vi "WriteBitDepth.vi"(8 "error in":errorcluster, 10 "BitDepth":u32, 11 "Image Reference In":T1) -> (0 "error out":errorcluster, 3 "Image Reference Out":T1)   [LabVIEW 2024, in "OpenLvVision_Image.lvlib" / "Management.lvlib"]
doc: "Sets number of bits per pixel, determining the range of representable colors or shades."
uses:
  Management.lvlib
  TypeDef/Image.ctl
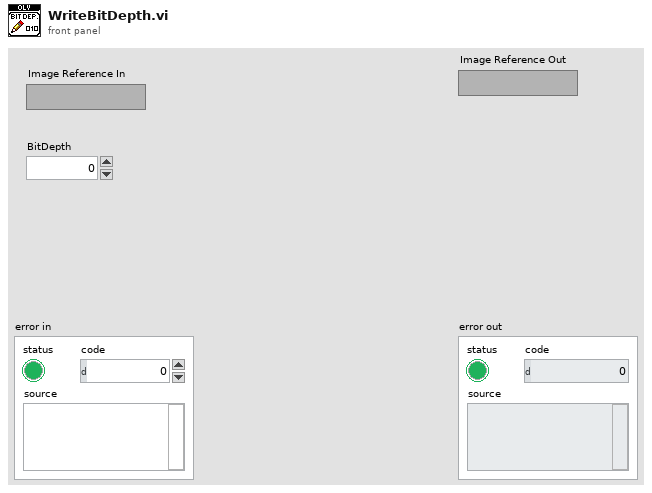
[diagram p1: front panel]
types:
  T1 = typedef "OpenLvVision_Image.lvlib/Management.lvlib/Image.ctl" = refnum<image>
  T2 = typedef "IMAQ Image.ctl" = refnum<image>
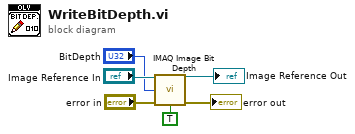
[diagram p0: block diagram]
diagram:
  n1 = call "IMAQ Image Bit Depth"("Image"="Image Reference In", "Bit Depth (0)"="BitDepth", "error in (no error)"="error in", "Get/Set Bit Depth? (Set)"=TRUE) -> ("Image Out"=→"Image Reference Out":T2, "error out"=→"error out":errorcluster)  [unwired: 9 in, 1 out]
